vi "Open Device.vi"() -> (0 "error out":errorcluster, 3 "HRF_Device out":refnum<class "HRF_Device.lvclass">)   [LabVIEW 2020, in "HRF_Device.lvclass"]
uses:
  HRF_Device.lvclass
  D:/work/HackRF/Labview Driver/NetHackrf.dll
  NetHackrf.dll
  HRF_Device.lvclass/HRF_Device.ctl
panel:
  out "reference out":refnum<k24>
  out "OpenDevice":refnum<k24>
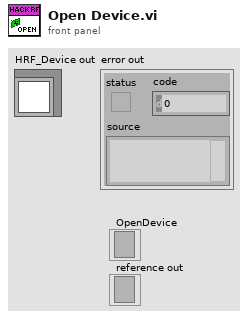
[diagram p1: front panel]
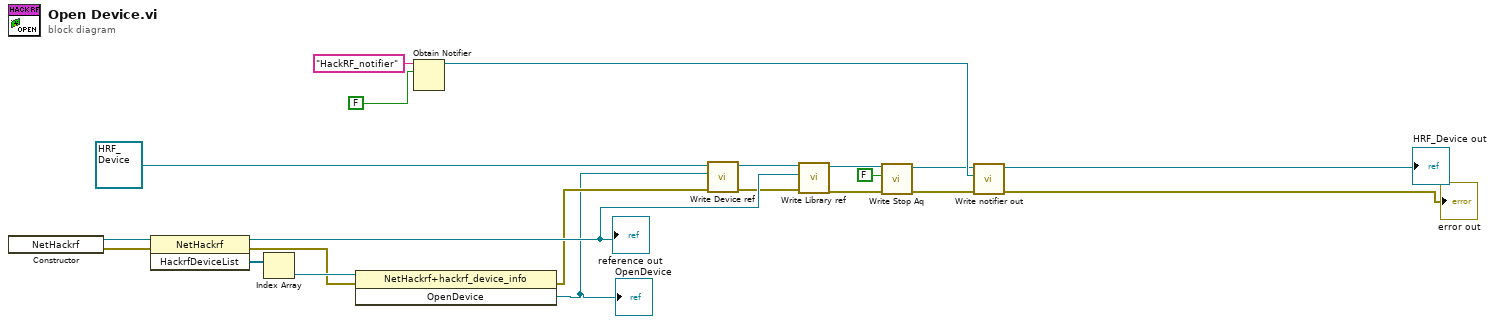
[diagram p0: block diagram]
diagram:
  n1 = constructor class="NetHackrf"() -> (reference out=w20:refnum<k24>, error out=w19:errorcluster)  [unwired: 3 in, 1 out]
  n2 = invoke class="NetHackrf" method="HackrfDeviceList"(reference=w20, error in=w19) -> (reference out=w14:refnum<k24>, error out=w17:errorcluster, "HackrfDeviceList"=w21:refnum<k24>[])  [unwired: 1 in]
  "reference out" <- w14
  n3 = Index Array(array=w21) -> (element=w18:refnum<k24>)  [unwired: 1 in]
  n4 = invoke class="NetHackrf+hackrf_device_info" method="OpenDevice"(reference=w18, error in=w17) -> (error out=w13:errorcluster, "OpenDevice"=w11:refnum<k24>)  [unwired: 1 in, 1 out]
  "OpenDevice" <- w11
  n5 = Obtain Notifier(name (unnamed)="HackRF_notifier", notification data type=FALSE) -> (notifier out=w5:refnum<notifier>)  [unwired: 2 in, 2 out]
  n6 = call "Write Device ref.vi"("error in (no error)"=w13, "Device ref"=w11, "HRF_Device in"=refnum<class "HRF_Device.lvclass"> refnum ("HRF_Device.lvclass")) -> ("error out"=w12:errorcluster, "HRF_Device out"=w15:refnum<class "HRF_Device.lvclass">)  [unwired: 7 in]
  n7 = call "Write Library ref.vi"("error in (no error)"=w12, "Library ref"=w14, "HRF_Device in"=w15) -> ("error out"=w10:errorcluster, "HRF_Device out"=w9:refnum<class "HRF_Device.lvclass">)  [unwired: 7 in]
  n8 = call "Write Stop Aq.vi"("error in (no error)"=w10, "Stop Aq"=FALSE, "HRF_Device in"=w9) -> ("error out"=w3:errorcluster, "HRF_Device out"=w4:refnum<class "HRF_Device.lvclass">)  [unwired: 7 in]
  n9 = call "Write notifier out.vi"("error in (no error)"=w3, "notifier out"=w5, "HRF_Device in"=w4) -> ("error out"=→"error out":errorcluster, "HRF_Device out"=→"HRF_Device out":refnum<class "HRF_Device.lvclass">)  [unwired: 7 in]
